vi "Teleop.vi"(10 "Match Info":T1={"Autonomous Elapsed Seconds"=0.0, "TeleOp Elapsed Seconds"=0.0, "Disabled Elapsed Seconds"=0.0, "Visited Autonomous"=FALSE, "Visited TeleOp"=FALSE, "Visited Disabled"=FALSE, "Autonomous Settings"={"Autonomous Style"=enum."Independent", "VI Refnum"=refnum}}, 11 "Call Context":T2) -> ()   [LabVIEW 2016]
doc: "This VI is called for each TeleOp packet received from the DS where the robot is not disabled. It is often used to read from the joysticks and update I/O or to update setpoints for timed control loops. It should complete and return within 20 milliseconds or it may miss DS packets."
uses:
  <vilib>/Rock Robotics/WPI/DriverStation/WPI_DriverStationDerivedRobotMode.ctl
  <vilib>/Rock Robotics/WPI/DriverStation/WPI_DriverStationMatch Info.ctl
  <vilib>/Rock Robotics/WPI/Utilities/WPI_GetSetVariantRefNum.vi
  <vilib>/Rock Robotics/Network Tables/NT Write Boolean Array.vi
  <vilib>/Rock Robotics/Network Tables/NT Write Numeric Array.vi
  <vilib>/Rock Robotics/Network Tables/NT Read Boolean.vi
  <vilib>/Rock Robotics/Network Tables/NT Read Number.vi
panel:
  out "Clamp Drive":dbl
  out "Which Button?":string
  out "Lift Bottom":dbl
  out "Lift Top":dbl
  out "Angle":dbl(knob) scale=0.0..360.0
  out "Sample Slider 0":dbl(slide) scale=0.0..5.0
  out "Sample Boolean 1":bool
  out "Sample Boolean 0":bool
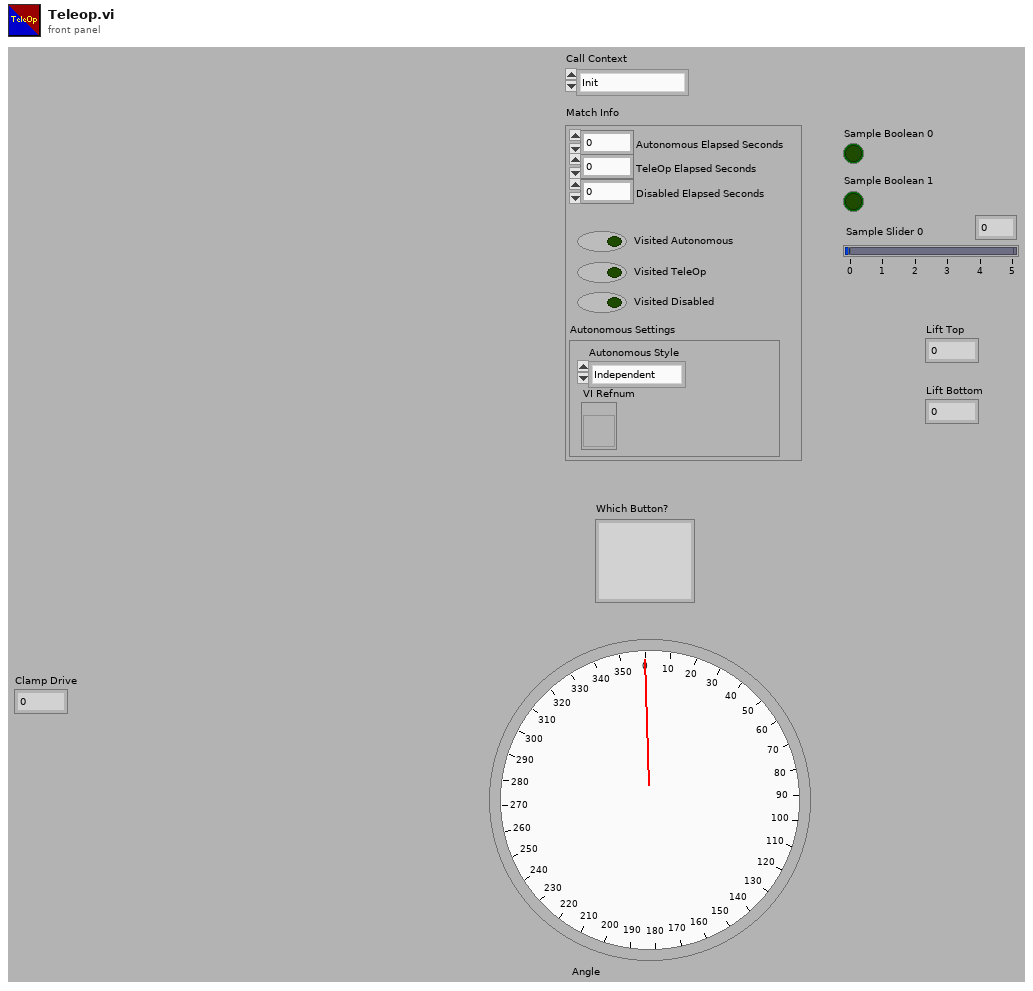
[diagram p1: front panel]
types:
  T1 = typedef "WPI_DriverStationMatch Info.ctl" = cluster{"Autonomous Elapsed Seconds":dbl, "TeleOp Elapsed Seconds":dbl, "Disabled Elapsed Seconds":dbl, "Visited Autonomous":bool, "Visited TeleOp":bool, "Visited Disabled":bool, "Autonomous Settings":cluster{"Autonomous Style":enum16{"Iterative", "Independent"}, "VI Refnum":refnum<vi>}}
  T2 = typedef "WPI_DriverStationDerivedRobotMode.ctl" = enum16{"Init", "Execute", "Stop"}
  T3 = typedef "WPI_MotorControlDeviceRef.ctl" = cluster{"DeviceStatus":errorcluster, "Type":T4, "PWM":cluster{"PWM Channel":T5, "DeadBand":T6}, "CAN":cluster{"Device Number":u8, "SetOutput VI Ref":variant, "GetOutput VI Ref":variant, "Enable VI Ref":variant, "Disable VI Ref":variant, "Data":variant}, "Invert":bool}
  T4 = typedef "WPI_MotorControlType.ctl" = enum16{"PWM", "CAN"}
  T5 = typedef "FPGA_DIOPWMChannel.ctl" = enum8{"PWM 0", "PWM 1", "PWM 2", "PWM 3", "PWM 4", "PWM 5", "PWM 6", "PWM 7", "PWM 8", "PWM 9", "PWM MXP 0", "PWM MXP 1", "PWM MXP 2", "PWM MXP 3", "PWM MXP 4", "PWM MXP 5", "PWM MXP 6", "PWM MXP 7", "PWM MXP 8", "PWM MXP 9", "Invalid"}
  T6 = typedef "WPI_PWMDeadband.ctl" = cluster{"Name":string, "maxPositivePwm":i32, "minPositivePwm":i32, "centerPwm":i32, "maxNegativePwm":i32, "minNegativePwm":i32, "angularRange":u16}
  T7 = typedef "WPI_GyroDevRef.ctl" = cluster{"DevStatus":errorcluster, "Analog Channel":T8, "Offset":dbl, "Gain (VoltsPerDegree/Second)":dbl, "Gyro Type":enum16{"Analog", "XRS450"}, "Handle":i32, "SPI Bus":T9, "Device Found":bool, "Sample Rate":dbl, "Calibrate On Open":bool}
  T8 = typedef "FPGA_AIChannel.ctl" = enum8{"AI 0", "AI 1", "AI 2", "AI 3", "AI MXP 0", "AI MXP 1", "AI MXP 2", "AI MXP 3", "Invalid"}
  T9 = typedef "spi_bus.ctl" = enum16{"SPI On-Board, CS0", "SPI On-Board, CS1", "SPI On-Board, CS2", "SPI On-Board, CS3", "SPI MXP", "Invalid"}
  T10 = typedef "WPI_RobotDriveDevRef.ctl" = cluster{"DevStatus":errorcluster, "Motors[]":T3[], "Square Inputs":bool, "Max Output":dbl}
  T11 = typedef "WPI_JoystickDevRef.ctl" = cluster{"Device":T12}
  T12 = typedef "WPI_JoystickDeviceEnum.ctl" = enum16{"USB 0", "USB 1", "USB 2", "USB 3", "USB 4", "USB 5"}
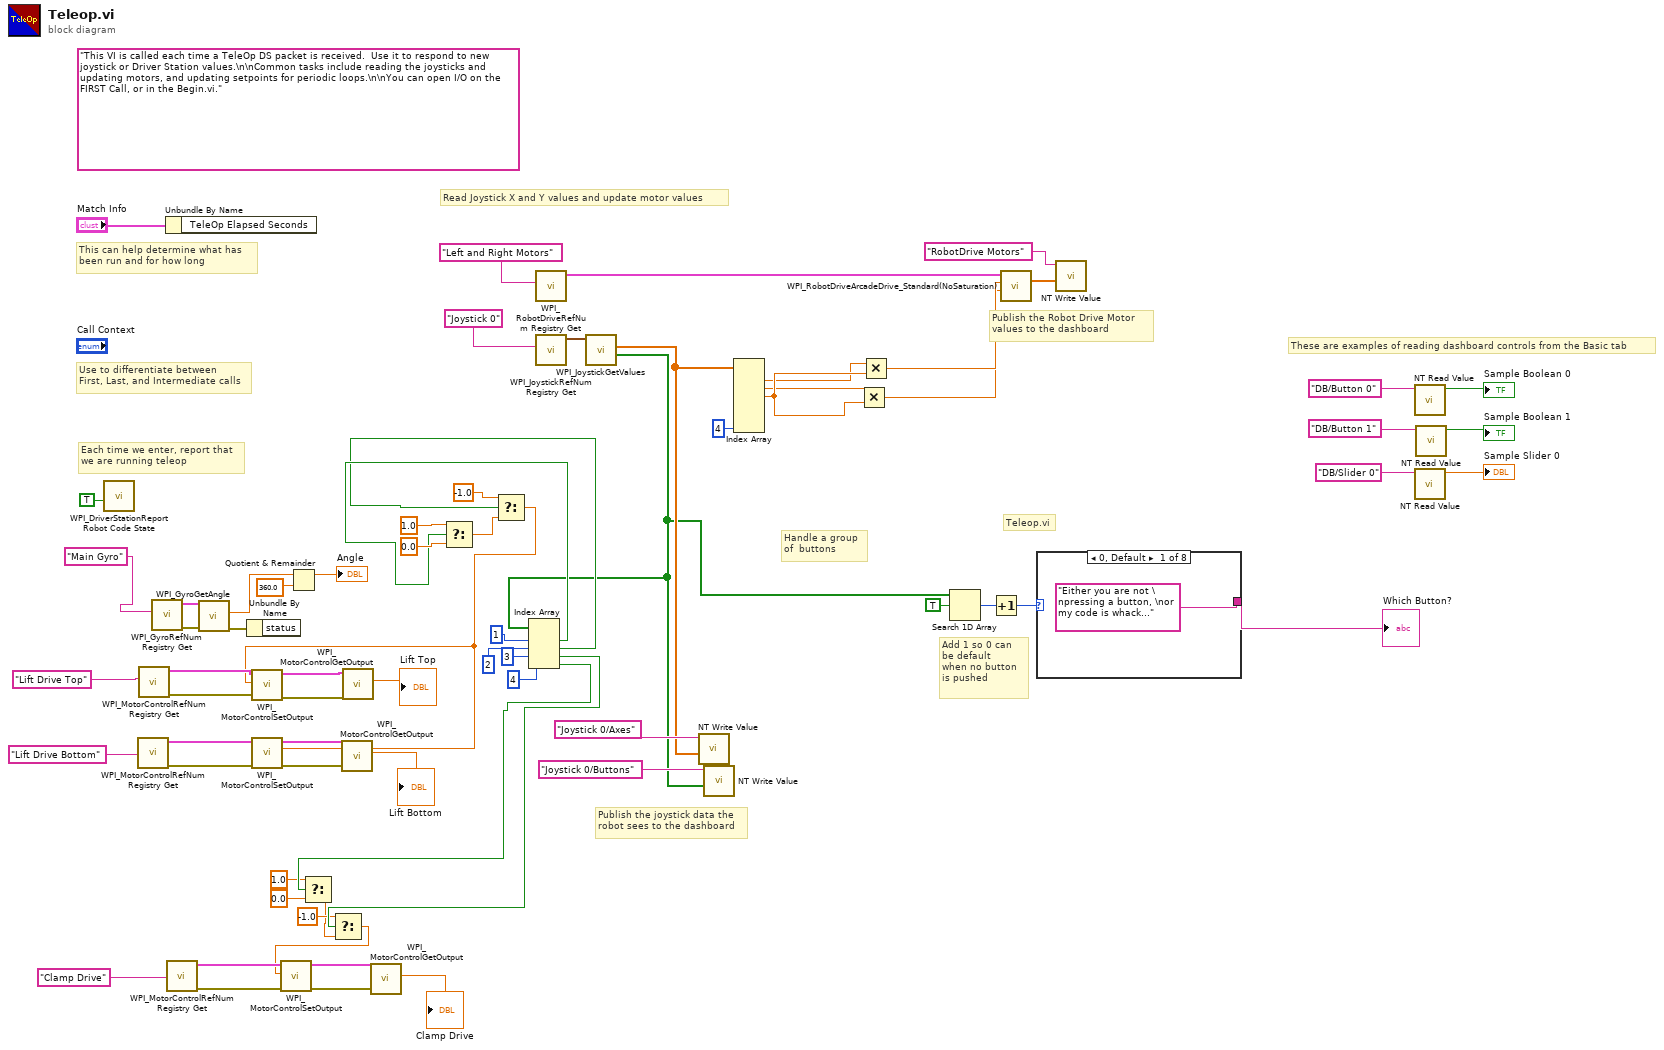
[diagram p0: block diagram]
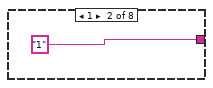
[diagram p2: hidden frame]
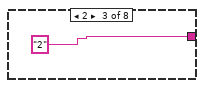
[diagram p3: hidden frame]
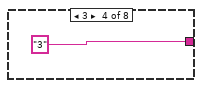
[diagram p4: hidden frame]
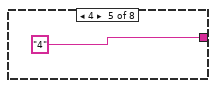
[diagram p5: hidden frame]
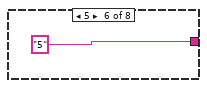
[diagram p6: hidden frame]
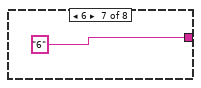
[diagram p7: hidden frame]
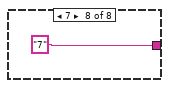
[diagram p8: hidden frame]
diagram:
  (unwired) "This VI is called each time a TeleOp DS packet is received.  Use it to respond to new joystick or Driver Station values.\n\nCommon tasks include reading the joysticks and updating motors, and updating setpoints for periodic loops.\n\nYou can open I/O on the FIRST Call, or in the Begin.vi."
  # "Teleop.vi"
  # "Handle a group\nof  buttons"
  # "Add 1 so 0 can\nbe default\nwhen no button\nis pushed"
  # "These are examples of reading dashboard controls from the Basic tab"
  # "Publish the Robot Drive Motor\nvalues to the dashboard"
  # "Publish the joystick data the\nrobot sees to the dashboard"
  # "Each time we enter, report that\nwe are running teleop"
  # "Use to differentiate between\nFirst, Last, and Intermediate calls"
  # "This can help determine what has\nbeen run and for how long"
  # "Read Joystick X and Y values and update motor values"
  n1 = call <vilib>:"WPI_DriverStationReport Robot Code State.vi"("TeleOp"=TRUE ("Autonomous")) -> ()  [unwired: 10 in, 1 out]
  n2 = call <vilib>:"WPI_MotorControlRefNum Registry Get.vi"("refnum name"="Lift Drive Bottom") -> ("error out"=w41:errorcluster, "MotorControlDevRef"=w37:T3)  [unwired: 9 in]
  n3 = call <vilib>:"WPI_MotorControlRefNum Registry Get.vi"("refnum name"="Lift Drive Top") -> ("error out"=w42:errorcluster, "MotorControlDevRef"=w38:T3)  [unwired: 9 in]
  n4 = call <vilib>:"WPI_GyroRefNum Registry Get.vi"("refnum name"="Main Gyro" ("Name")) -> ("error out"=w45:errorcluster, "GyroDevRef"=w44:T7)  [unwired: 9 in]
  n5 = Unbundle By Name("Match Info") -> ()  [unwired: 1 out]
  n6 = call <vilib>:"WPI_MotorControlRefNum Registry Get.vi"("refnum name"="Clamp Drive") -> ("error out"=w15:errorcluster, "MotorControlDevRef"=w13:T3)  [unwired: 9 in]
  n7 = call <vilib>:"WPI_GyroGetAngle.vi"("error in"=w45, "GyroDevRef"=w44) -> ("error out"=w46:errorcluster, "Angle"=w47:dbl)  [unwired: 5 in, 3 out]
  n8 = Unbundle By Name(w46) -> ()  [unwired: 1 out]
  n9 = Quotient & Remainder(x=w47, y=360.0) -> (x-y*floor(x/y)=→"Angle":dbl)  [unwired: 1 out]
  n10 = call <vilib>:"WPI_RobotDriveRefNum Registry Get.vi"("refnum name"="Left and Right Motors") -> ("RobotDriveDevRef"=w69:T10)  [unwired: 1 in, 9 out]
  n11 = call <vilib>:"WPI_JoystickRefNum Registry Get.vi"("refnum name"="Joystick 0") -> ("JoystickDevRef"=w68:T11)  [unwired: 1 in, 9 out]
  n12 = call <vilib>:"WPI_JoystickGetValues.vi"("JoystickDevRef"=w68) -> ("Buttons"=w17:bool[], "Axes"=w64:dbl[])  [unwired: 6 in, 3 out]
  n13 = Index Array "Index Array"(array=w17, index #1=1 ("index"), index #2=2 ("index"), index #3=3 ("index"), index #4=4 ("index")) -> (element #1=w25:bool, element #2=w22:bool, element #3=w7:bool, element #4=w6:bool)
  n14 = Select(t=1.0, s=w6, f=0.0) -> (s? t:f=w2:dbl)
  n15 = Select(t=-1.0, s=w7, f=w2) -> (s? t:f=w1:dbl)
  n16 = call <vilib>:"WPI_MotorControlSetOutput.vi"("error in (no error)"=w15, "Output"=w1, "MotorControlDevRef"=w13) -> ("error out"=w12:errorcluster, "MotorControlDevRef"=w14:T3)  [unwired: 6 in, 1 out]
  n17 = call <vilib>:"WPI_MotorControlGetOutput.vi"("error in"=w12, "MotorControlDevRef"=w14) -> ("Output"=→"Clamp Drive":dbl)  [unwired: 7 in, 2 out]
  n18 = Select(t=1.0, s=w25, f=0.0) -> (s? t:f=w21:dbl)
  n19 = Select(t=-1.0, s=w22, f=w21) -> (s? t:f=w23:dbl)
  n20 = call <vilib>:"WPI_MotorControlSetOutput.vi"("error in (no error)"=w42, "Output"=w23, "MotorControlDevRef"=w38) -> ("error out"=w36:errorcluster, "MotorControlDevRef"=w39:T3)  [unwired: 6 in, 1 out]
  n21 = call <vilib>:"WPI_MotorControlSetOutput.vi"("error in (no error)"=w41, "Output"=w23, "MotorControlDevRef"=w37) -> ("error out"=w35:errorcluster, "MotorControlDevRef"=w40:T3)  [unwired: 6 in, 1 out]
  n22 = call <vilib>:"WPI_MotorControlGetOutput.vi"("error in"=w35, "MotorControlDevRef"=w40) -> ("Output"=→"Lift Bottom":dbl)  [unwired: 7 in, 2 out]
  n23 = call <vilib>:"WPI_MotorControlGetOutput.vi"("error in"=w36, "MotorControlDevRef"=w39) -> ("Output"=→"Lift Top":dbl)  [unwired: 7 in, 2 out]
  n24 = call-poly <vilib>:"NT Write Value.vi"("Numeric Array"=w64, "Name"="Joystick 0/Axes") -> ()  [unwired: 9 in, 1 out]
  n25 = call-poly <vilib>:"NT Write Value.vi"("Boolean Array"=w17, "Name"="Joystick 0/Buttons") -> ()  [unwired: 9 in, 1 out]
  n26 = Index Array(array=w64, index #7=4 ("index")) -> (element #1=w52:dbl, element #2=w53:dbl, element #3=w54:dbl)  [unwired: 6 in, 4 out]
  n27 = Multiply(x=w53, y=w54) -> (x*y=w50:dbl)
  n28 = Multiply(x=w52, y=w54) -> (x*y=w51:dbl)
  n29 = Search 1D Array(1D array=w17, element=TRUE) -> (index of element=w19:i32)  [unwired: 1 in]
  n30 = Increment(x=w19) -> (x+1=w18:i32)
  n31 = call <vilib>:"WPI_RobotDriveArcadeDrive_Standard(NoSaturation).vi"("Y axis value"=w50, "X axis value"=w51, "RobotDriveDevRef"=w69) -> ("Motor Values"=w57:dbl[])  [unwired: 1 in, 7 out]
  n32 = case shown="0, Default" w18 {
    tunnel: ["Either you are not \npressing a button, \nor my code is whack..." "1" "2" "3" "4" "5" "6" "7"] -> w16
    frame 0, Default {
    }
    frame 1 {
    }
    frame 2 {
    }
    frame 3 {
    }
    frame 4 {
    }
    frame 5 {
    }
    frame 6 {
    }
    frame 7 {
    }
  }
  "Which Button?" <- w16
  n33 = call-poly <vilib>:"NT Write Value.vi"("Numeric Array"=w57, "Name"="RobotDrive Motors") -> ()  [unwired: 9 in, 1 out]
  n34 = call-poly <vilib>:"NT Read Value.vi"("Name"="DB/Button 0" ("refnum name")) -> ("Boolean"=→"Sample Boolean 0":bool)  [unwired: 9 in, 1 out]
  n35 = call-poly <vilib>:"NT Read Value.vi"("Name"="DB/Slider 0" ("refnum name")) -> ("Numeric"=→"Sample Slider 0":dbl)  [unwired: 9 in, 1 out]
  n36 = call-poly <vilib>:"NT Read Value.vi"("Name"="DB/Button 1" ("refnum name")) -> ("Boolean"=→"Sample Boolean 1":bool)  [unwired: 9 in, 1 out]
